vi "SysInfo-Get Experiment VIs Subfolder.vi"(4 "subfolder":string) -> (1 "full path":path)   [LabVIEW 2020]
uses:
  <vilib>/Utility/sysdir.llb/System Directory Type.ctl
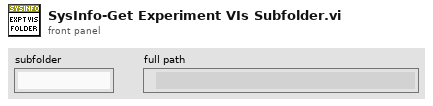
[diagram p1: front panel]
types:
  T1 = typedef "System Directory Type.ctl" = i32
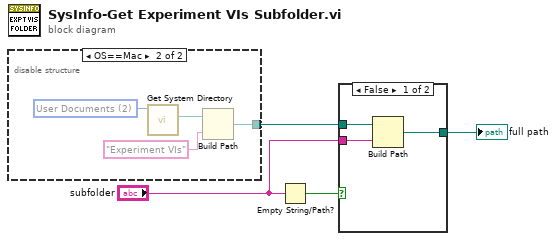
[diagram p0: block diagram]
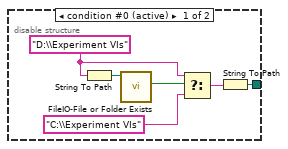
[diagram p2: hidden frame]
diagram:
  n1 = disable-structure shown="OS==Mac" {
    disable-tunnel: [w5 w11] -> w4
    frame condition #0 (active) {
      w8 = "D:\\Experiment VIs" ("wcPath")
      n2 = String To Path(string=w8) -> (path=w10:path)
      n3 = call "FileIO-File or Folder Exists.vi"("path"=w10) -> ("Directory?"=w9:bool)  [unwired: 7 in, 3 out]
      n4 = Select(t=w8, s=w9, f="C:\\Experiment VIs" ("wcPath")) -> (s? t:f=w6:string)
      n5 = String To Path(string=w6) -> (path=w5:path)
    }
    frame condition #1 {
      w12 = T1 2 items=["User Home"=0, "User Desktop"=1, "User Documents"=2, "User Application Data"=3, "User Preferences"=4, "User Temporary"=5, "Public Documents"=6, "Public Application Data"=7, "Public Preferences"=8, "Public Cache"=13, "System Core Libraries"=9, "System Installed Libraries"=10, "Application Files"=11, "Boot Volume Root"=12] ("system directory type")
      n6 = call <vilib>:"Get System Directory.vi"("system directory type"=w12) -> ("system directory"=w13:path)  [unwired: 10 in]
      n7 = Build Path(base path=w13, name or relative path="Experiment VIs") -> (appended path=w11:path)
    }
  }
  n8 = Empty String/Path?(string/path="subfolder") -> (empty?=w1:bool)
  n9 = case shown="False" w1 {
    tunnel: w4 -> [w17 w18]
    tunnel: [w16 w18] -> w3
    tunnel: "subfolder" -> [w15 _]
    frame False {
      n10 = Build Path(base path=w17, name or relative path=w15) -> (appended path=w16:path)
    }
    frame True {
    }
  }
  "full path" <- w3
